vi "Request Data JSON.vi"(8 "error in (no error)":errorcluster, 11 "Sleep in":refnum<class "Sleep.lvclass">) -> (0 "error out":errorcluster, 2 "Request Data JSON":string, 3 "Sleep out":refnum<class "Sleep.lvclass">)   [LabVIEW 2022 SP3, in "obs-websocket-lv.lvlib" / "Sleep.lvclass"]
uses:
  Sleep.lvclass
  Sleep.lvclass/Sleep.ctl
  <vilib>/IlluminatedG/lv-web-crypto/lv-json/JSON/JSON.lvlib
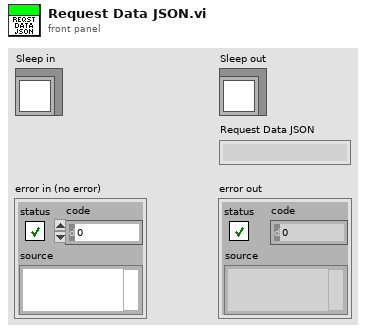
[diagram p1: front panel]
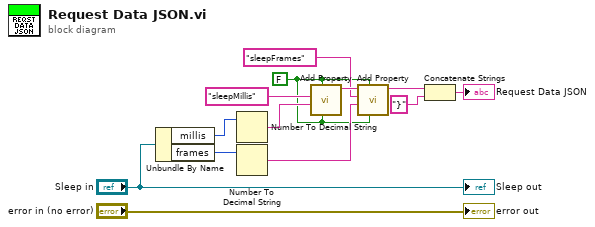
[diagram p0: block diagram]
diagram:
  w1 = FALSE ("Include Empty?")
  n1 = Unbundle By Name("Sleep in") -> ("millis"=w11:u16, "frames"=w10:u16)
  n2 = Number To Decimal String(number=w11) -> (decimal integer string=w9:string)  [unwired: 1 in]
  n3 = Number To Decimal String(number=w10) -> (decimal integer string=w5:string)  [unwired: 1 in]
  n4 = call <vilib>:"Add Property.vi"("String?"=w1, "Include Empty?"=w1, "Value"=w9, "Property Name"="sleepMillis") -> ("String out"=w7:string)  [unwired: 7 in]
  n5 = call <vilib>:"Add Property.vi"("String?"=w1, "Include Empty?"=w1, "Value"=w5, "Property Name"="sleepFrames", "String In"=w7) -> ("String out"=w4:string)  [unwired: 6 in]
  n6 = Concatenate Strings(w4, "}" ("string")) -> (→"Request Data JSON":string)
  "error out" <- "error in (no error)"
  "Sleep out" <- "Sleep in"
